vi "Append Info to Error.vi"(8 "error in (no error)":errorcluster, 11 "additional info":string) -> (0 "error out":errorcluster)   [LabVIEW 2020, in "NI_SSH.lvlib"]
uses:
  <vilib>/net/SSH/NI_SSH.lvlib
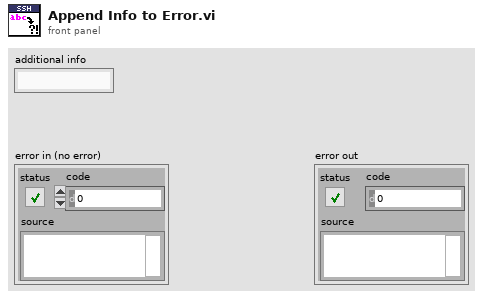
[diagram p1: front panel]
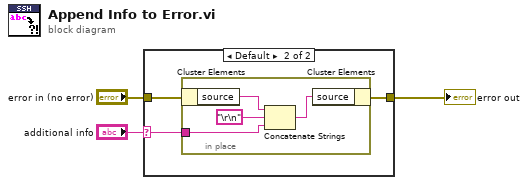
[diagram p0: block diagram]
diagram:
  n1 = case shown="Default" "additional info" {
    selector: "additional info" -> [_ w5]
    tunnel: [w4 w7] -> w3
    tunnel: "error in (no error)" -> [w4 w6]
    frame "" {
    }
    frame Default {
      n2 = in-place {
        in-place-border: w5 -> [w9]
        n3 = in-place-cluster #1(w6) -> ("source"=w11:string)
        n4 = Concatenate Strings(w11, "\r\n", w9) -> (w8:string)
        n5 = in-place-cluster #1("source"=w8) -> (w7:errorcluster)
      }
    }
  }
  "error out" <- w3
